vi "Test Tree UI.vi"() -> ()   [LabVIEW 2020, in "Sequencer with Output Values.lvlib" / "Sequencer with Output Values.lvclass"]
uses:
  Sequencer with Output Values.lvclass
  Params.ctl
  Step Settings.ctl
  Tree Manager/Tree Manager Mode.ctl
panel:
  out "Applied Settings":T1={"Step Values"=[], "Only Execute When Test Running"=TRUE, "Reset Sequence When Test Starts"=TRUE, "Current Sequence ID"=0, "Total Iterations"=0, "Current Step Start Timestamp"=0.0, "Number of Sequence Steps"=0, "Num of Analog Channels"=0, "Num of Digital Channels"=0, "Delay Before Starting Sequence"=0.0, "Show UI"=FALSE, "Time Remaining"=0.0, "Test Running"=FALSE, "Pause Timestamp"=0.0}
  in  "Show":bool
  in  "stop":bool
  out "Current Settings JSON String":string
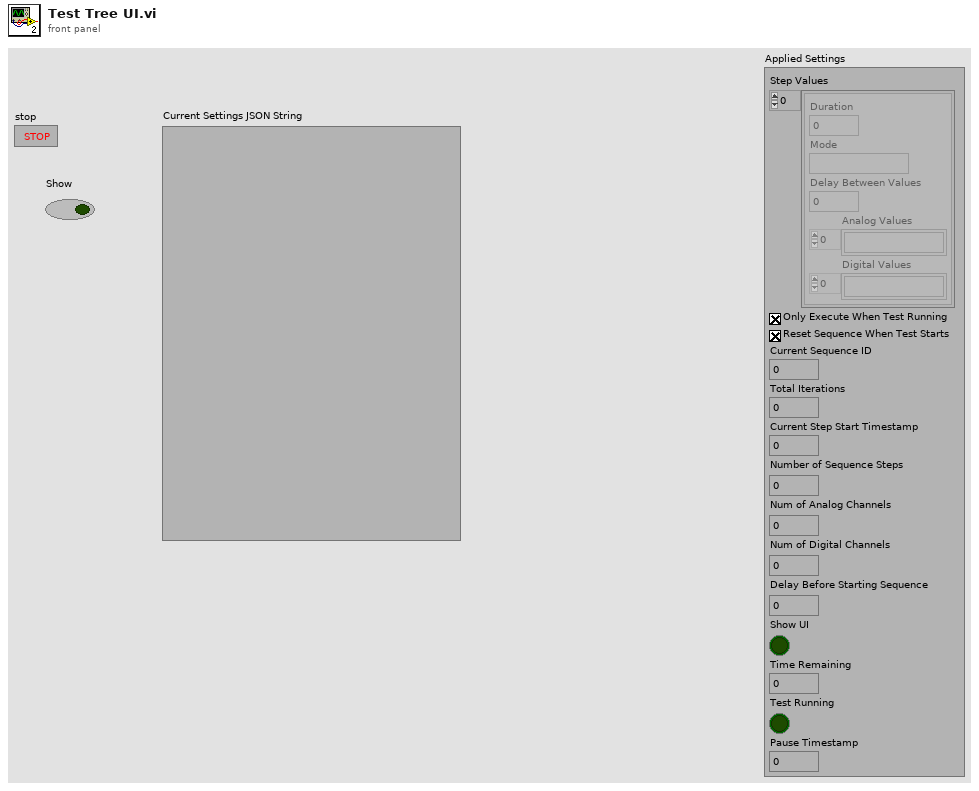
[diagram p1: front panel]
types:
  T1 = typedef "Sequencer with Output Values.lvlib/Sequencer with Output Values.lvclass/Params.ctl" = cluster{"Step Values":T2[], "Only Execute When Test Running":bool, "Reset Sequence When Test Starts":bool, "Current Sequence ID":u32, "Total Iterations":u32, "Current Step Start Timestamp":dbl, "Number of Sequence Steps":i32, "Num of Analog Channels":i32, "Num of Digital Channels":i32, "Delay Before Starting Sequence":dbl, "Show UI":bool, "Time Remaining":dbl, "Test Running":bool, "Pause Timestamp":dbl}
  T2 = typedef "Sequencer with Output Values.lvlib/Sequencer with Output Values.lvclass/Step Settings.ctl" = cluster{"Duration":dbl, "Mode":string, "Delay Between Values":dbl, "Analog Values":string[], "Digital Values":string[]}
  T3 = typedef "Sequencer with Output Values.lvlib/Sequencer with Output Values.lvclass/Tree Manager Mode.ctl" = enum16{"Init", "Tree Change", "Value Change", "Close"}
  T4 = enum32{"Invalid", "Standard", "Closed", "Hidden", "Minimized", "Maximized"}
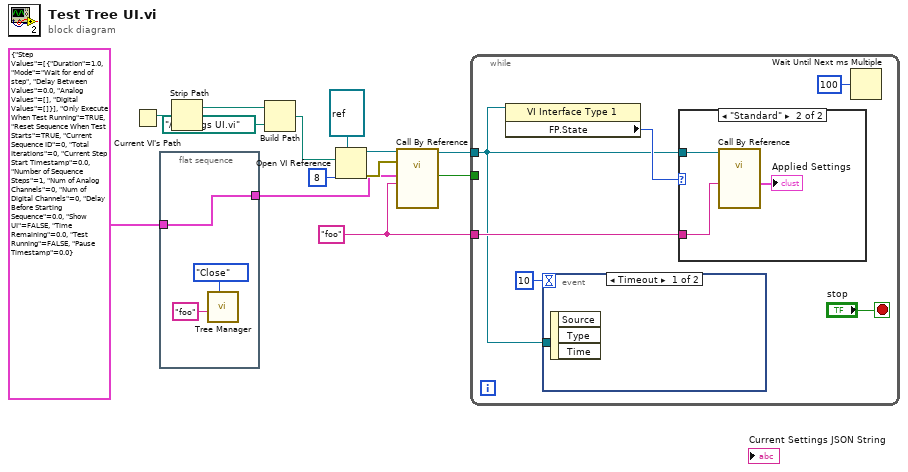
[diagram p0: block diagram]
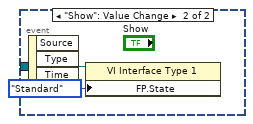
[diagram p2: hidden frame]
diagram:
  w10 = "foo" ("Alias")
  n1 = Current VI's Path() -> (path=w5:path)
  n2 = flat-sequence {
    tunnel: [w14] -> w1
    tunnel: T1 {"Step Values"=[{"Duration"=1.0, "Mode"="Wait for end of step", "Delay Between Values"=0.0, "Analog Values"=[], "Digital Values"=[]}], "Only Execute When Test Running"=TRUE, "Reset Sequence When Test Starts"=TRUE, "Current Sequence ID"=0, "Total Iterations"=0, "Current Step Start Timestamp"=0.0, "Number of Sequence Steps"=1, "Num of Analog Channels"=0, "Num of Digital Channels"=0, "Delay Before Starting Sequence"=0.0, "Show UI"=FALSE, "Time Remaining"=0.0, "Test Running"=FALSE, "Pause Timestamp"=0.0} ("Settings In") -> [w14]
    frame #0 {
      n3 = call "Tree Manager.vi"("Mode"=Tree_Manager_Mode."Close", "Alias"="foo") -> ()  [unwired: 9 in, 1 out]
    }
  }
  n4 = Strip Path(path=w5) -> (stripped path=w4:path)  [unwired: 1 out]
  n5 = Build Path(base path=w4, name or relative path=path "../Settings UI.vi") -> (appended path=w2:path)
  n6 = Open VI Reference(type specifier VI Refnum (for type only)=refnum<vi> refnum, vi path=w2, options=8) -> (vi reference=w7:refnum<vi>, error out=w11:errorcluster)  [unwired: 3 in]
  n7 = call-by-ref "?"(reference=w7, error in=w11, "Alias"=w10, "Init Settings In"=w1) -> (reference out=w8:refnum<vi>, "Show UI"=w9:bool)  [unwired: 8 in, 2 out]
  n8 = while {
    tunnel: w10 -> [w20]
    tunnel: w9 -> [_]
    tunnel: w8 -> [w17]
    stop <- "stop" stop-if-true
    n9 = property class="VI Interface Type 1"(reference=w17) -> ("FP.State"=w19:T4)  [unwired: 1 in, 2 out]
    n10 = event shown="[0] Timeout" {
      selector: _ -> [_ _]
      dyn-events: _ -> [_ _]
      timeout: 10 -> [_ _]
      tunnel: w17 -> [_ w24]
      event Timeout {
        n11 = event-data() -> ()  [unwired: 1 in, 3 out]
      }
      event "Show": Value Change {
        n12 = event-data() -> ()  [unwired: 1 in, 3 out]
        n13 = property class="VI Interface Type 1"(reference=w24, "FP.State"=T4."Standard" ("Front Panel Window:State")) -> ()  [unwired: 1 in, 2 out]
      }
    }
    n14 = case shown="\"Standard\"" w19 {
      tunnel: w20 -> [_ w27]
      tunnel: w17 -> [_ w26]
      frame "Invalid", Default {
      }
      frame "Standard" {
        n15 = call-by-ref "?"(reference=w26, "Alias"=w27) -> ("Applied Settings"=→"Applied Settings":T1)  [unwired: 10 in, 3 out]
      }
    }
    n16 = Wait Until Next ms Multiple(millisecond multiple=u32 100) -> ()  [unwired: 1 out]
  }
